vi "test_OneSessTwoPinOneInstrOneSiteReservation_VISAGetConnections1PinMConnections_ReturnsTwoConnections.vi"(8 "error in":errorcluster) -> (0 "error out":errorcluster, 2 "result":string, 3 "pass":bool)   [LabVIEW 2020, in "MeasurementServerTests.lvlib"]
uses:
  MeasurementServerTests.lvlib
  Runtime/Measurements/Measurement Plugin Session Management V1/Session Reservation/Connection.ctl
  Runtime/Measurements/Measurement Plugin Session Management V1/Session Reservation/Session Reservation.lvclass
  03fc85e1-696b-4ece-a78b-f41470766ac0.vi
  a536e905-e99b-4ce6-9f7b-add65bd26abc.vi
  Runtime/MeasurementLink VISA/MeasurementLink VISA.lvlib
  Runtime/MeasurementLink VISA/Get Connections - 1Pin MConn.vi
  Runtime/MeasurementLink VISA/Connection with Session.ctl
  88858efc-9bbe-47cb-856b-78f33cdfecc8.vi
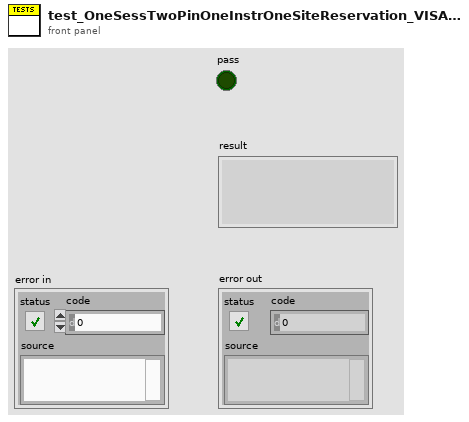
[diagram p1: front panel]
types:
  T1 = typedef "Measurement Plugin Session Management V1.lvlib/Session Reservation.lvclass/Connection.ctl" = cluster{"pin or relay name":string, "site":i32, "instrument type id":string, "channel":string}
  T2 = typedef "MeasurementLink VISA.lvlib/Connection with Session.ctl" = cluster{"connection":T1, "session":refnum<visa-resource-name>}
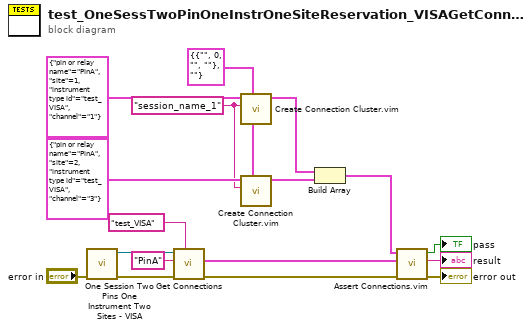
[diagram p0: block diagram]
diagram:
  w10 = T2 {"connection"={"pin or relay name"="", "site"=0, "instrument type id"="", "channel"=""}, "session"=""} ("niDCPower connection")
  w9 = "session_name_1" ("session in")
  n1 = call "One Session Two Pins One Instrument Two Sites - VISA.vi"("error in"="error in") -> ("error out"=w4:errorcluster, "session reservation out"=w5:refnum<class "Session Reservation.lvclass">)  [unwired: 9 in]
  n2 = call-poly "Get Connections.vi"("instrument type id"="test_VISA", "error in"=w4, "pin or relay name"="PinA", "session reservation in"=w5) -> ("error out"=w2:errorcluster, "connections"=w17:T2[])  [unwired: 5 in, 1 out]
  n3 = call "Create Connection Cluster.vim"("connection type"=w10, "session in"=w9, "hardware independent connection in"=T1 {"pin or relay name"="PinA", "site"=1, "instrument type id"="test_VISA", "channel"="1"} ("connection")) -> ("connection out"=w8:T2)  [unwired: 8 in]
  n4 = call "Create Connection Cluster.vim"("connection type"=w10, "session in"=w9, "hardware independent connection in"=T1 {"pin or relay name"="PinA", "site"=2, "instrument type id"="test_VISA", "channel"="3"} ("connection")) -> ("connection out"=w7:T2)  [unwired: 8 in]
  n5 = Build Array(w8, w7) -> (w6:T2[])
  n6 = call "Assert Connections.vim"("error in"=w2, "actual connections"=w17, "expected connections"=w6) -> ("error out"=→"error out":errorcluster, "result"=→"result":string, "pass"=→"pass":bool)  [unwired: 6 in]
